vi "CTRE_Phoenix_CANCoder_GetAbsolutePosition.vi"(8 "error in":errorcluster, 11 "CTRE_CANcoder_DeviceRef":T1) -> (0 "error out":errorcluster, 2 "Absolute Position":dbl format="%.2f", 3 "CTRE_CANcoder_DeviceRef":T1)   [LabVIEW 2019]
doc: "Returns the absolute position of the CANcoder."
uses:
  <vilib>/Rock Robotics/WPI/ThirdParty/Phoenix-LabVIEW/CANCoder/Controls/CTRE_Phoenix_CANcoder_DeviceRef.ctl
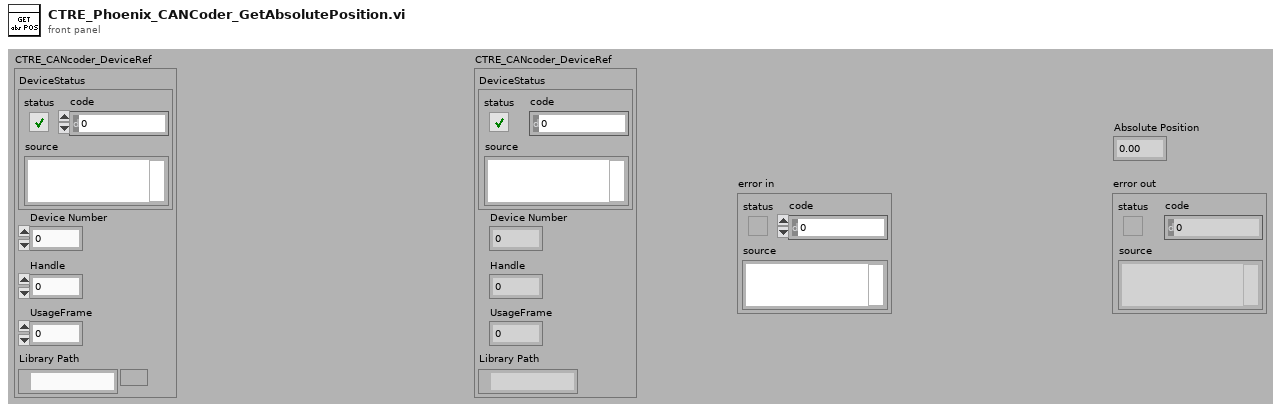
[diagram p1: front panel]
types:
  T1 = typedef "CTRE_Phoenix_CANcoder_DeviceRef.ctl" = cluster{"DeviceStatus":errorcluster, "Device Number":u8, "Handle":u64, "UsageFrame":u32, "Library Path":path}
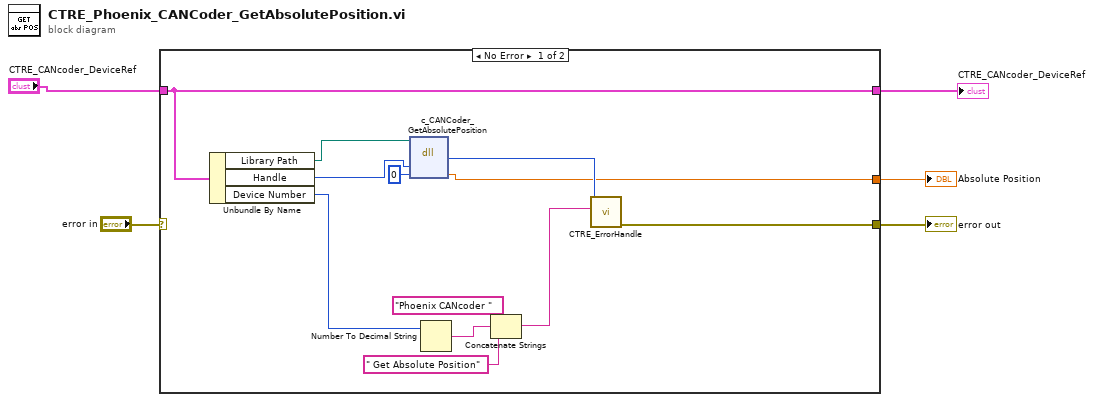
[diagram p0: block diagram]
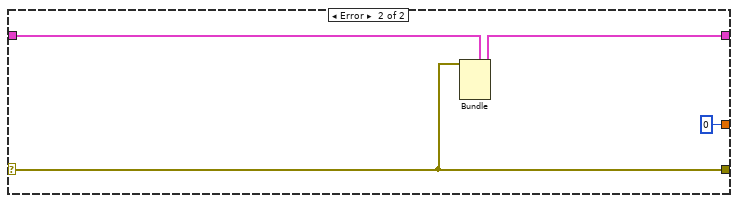
[diagram p2: hidden frame]
diagram:
  n1 = case shown="No Error" "error in" {
    selector: "error in" -> [_ w20]
    tunnel: "CTRE_CANcoder_DeviceRef" -> [w9 w21]
    tunnel: [w16 w20] -> w5
    tunnel: [w9 w19] -> w1
    tunnel: [w10 0 ("percentOutput")] -> w3
    frame No Error {
      n2 = Unbundle By Name(w9) -> ("Library Path"=w7:path, "Handle"=w6:u64, "Device Number"=w8:u8)
      n3 = dll-call lib="?" fn="c_CANCoder_GetAbsolutePosition"(path in=w7, "handle"=w6, "absPosition"=0 ("appliedThrottle")) -> ("return type"=w12:i32, "absPosition"=w10:dbl)  [unwired: 3 in, 2 out]
      n4 = Number To Decimal String(number=w8) -> (decimal integer string=w14:string)  [unwired: 1 in]
      n5 = Concatenate Strings("Phoenix CANcoder " ("string"), w14, " Get Absolute Position" ("string")) -> (w11:string)
      n6 = call <vilib>:"CTRE_ErrorHandle.vi"("origin"=w11, "code"=w12) -> ("error out"=w16:errorcluster)  [unwired: 9 in]
    }
    frame Error {
      n7 = Bundle(cluster=w21, "DeviceStatus"=w20) -> (w19:T1)  [unwired: 4 in]
    }
  }
  "Absolute Position" <- w3
  "error out" <- w5
  "CTRE_CANcoder_DeviceRef" <- w1
